vi "TestStand, Set Step Data, Boolean.vi"(8 "error in":errorcluster, 10 "Result (F)":bool caption="Result", 11 "Sequence Context":refnum<k7>) -> (0 "error out":errorcluster, 3 "Sequence Context Out":refnum<k7>)   [LabVIEW 2010]
doc: "Transfers measurement results to the default TestStand Boolean Test data element (RunState.Step.Result.PassFail)."
uses:
  <vilib>/addons/TestStand/_TSUtility.llb/TestStand - Set Property Value (Boolean).vi
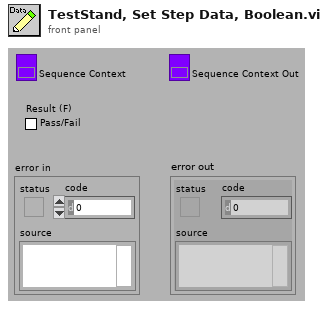
[diagram p1: front panel]
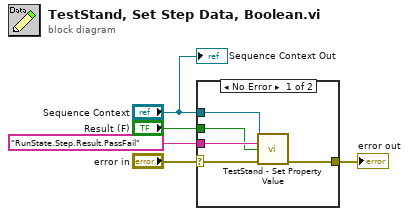
[diagram p0: block diagram]
diagram:
  n1 = case shown="No Error" "error in" {
    selector: "error in" -> [w8 w11]
    tunnel: [w9 w11] -> w5
    tunnel: "Sequence Context" -> [w10 _]
    tunnel: "RunState.Step.Result.PassFail" ("suffix") -> [w7 _]
    tunnel: "Result (F)" -> [w6 _]
    frame No Error {
      n2 = call-poly <vilib>:"TestStand - Set Property Value.vi"("Sequence Context In"=w10, "Lookup String"=w7, "New Value"=w6, "error in (no error)"=w8) -> ("error out"=w9:errorcluster)  [unwired: 10 in, 1 out]
    }
    frame Error {
    }
  }
  "error out" <- w5
  "Sequence Context Out" <- "Sequence Context"
